vi "All Channel Data.vi"(8 "Error In":errorcluster, 11 "Adc Convertor In":refnum<class "Adc Convertor.lvclass">) -> (0 "Error Out":errorcluster, 3 "Adc Convertor Out":refnum<class "Adc Convertor.lvclass">)   [LabVIEW 2021, in "Adc Convertor.lvclass"]
doc: "This VI gets the all channel data parallely."
uses:
  Adc Convertor.lvclass
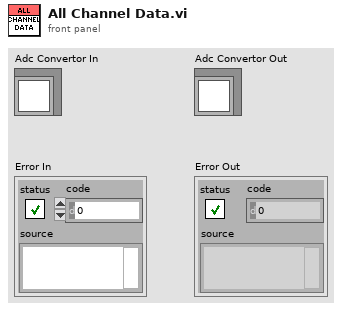
[diagram p1: front panel]
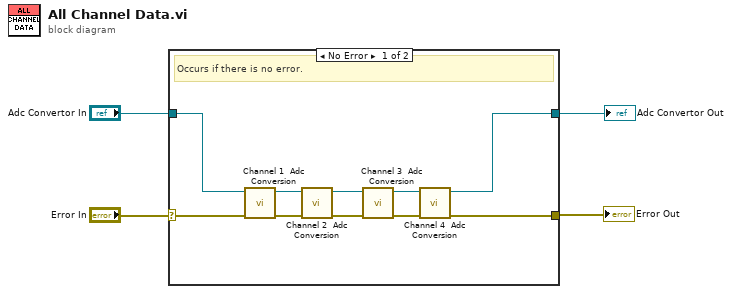
[diagram p0: block diagram]
diagram:
  n1 = case shown="No Error" "Error In" {
    selector: "Error In" -> [w13 w16]
    tunnel: [w6 w16] -> w3
    tunnel: [w5 w15] -> w1
    tunnel: "Adc Convertor In" -> [w14 w15]
    frame No Error {
      # "Occurs if there is no error."
      n2 = call "Channel 1  Adc Conversion.vi"("Error In"=w13, "Adc Convertor In"=w14) -> ("Error Out"=w9:errorcluster, "Adc Convertor Out"=w12:refnum<class "Adc Convertor.lvclass">)  [unwired: 8 in]
      n3 = call "Channel 2  Adc Conversion.vi"("Error In"=w9, "Adc Convertor In"=w12) -> ("Error Out"=w8:errorcluster, "Adc Convertor Out"=w11:refnum<class "Adc Convertor.lvclass">)  [unwired: 8 in]
      n4 = call "Channel 3  Adc Conversion.vi"("Error In"=w8, "Adc Convertor In"=w11) -> ("Error Out"=w7:errorcluster, "Adc Convertor Out"=w10:refnum<class "Adc Convertor.lvclass">)  [unwired: 8 in]
      n5 = call "Channel 4  Adc Conversion.vi"("Error In"=w7, "Adc Convertor In"=w10) -> ("Error Out"=w6:errorcluster, "Adc Convertor Out"=w5:refnum<class "Adc Convertor.lvclass">)  [unwired: 8 in]
    }
    frame Error {
      # "Occurs if there is any error."
    }
  }
  "Error Out" <- w3
  "Adc Convertor Out" <- w1
